vi "Signal Waiting VIs.vi"(4 "Error In":errorcluster) -> (0 "Error Out":errorcluster)   [LabVIEW 2015, in "not_Launch Completed.lvlib"]
uses:
  not_Launch Completed.lvlib
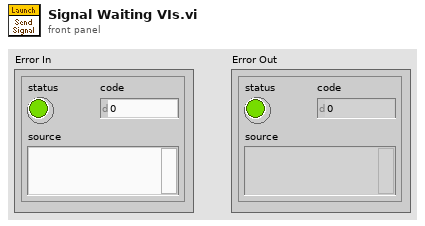
[diagram p1: front panel]
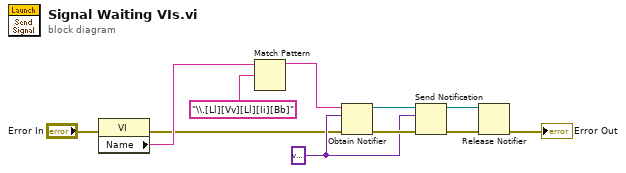
[diagram p0: block diagram]
diagram:
  w7 = variant ("element data type")
  n1 = property class="VI"(error in="Error In") -> (error out=w4:errorcluster, "Name"=w6:string)  [unwired: 1 in, 1 out]
  n2 = Match Pattern(string=w6, regular expression="\\.[Ll][Vv][Ll][Ii][Bb]") -> (before substring=w3:string)  [unwired: 1 in, 3 out]
  n3 = Obtain Notifier(name (unnamed)=w3, notification data type=w7, error in (no error)=w4) -> (notifier out=w10:refnum<notifier>, error out=w11:errorcluster)  [unwired: 1 in, 1 out]
  n4 = Send Notification(notification=w7, notifier=w10, error in (no error)=w11) -> (notifier out=w9:refnum<notifier>, error out=w8:errorcluster)
  n5 = Release Notifier(notifier=w9, error in (no error)=w8) -> (error out=→"Error Out":errorcluster)  [unwired: 1 in, 2 out]
